vi "_allan_Variance_Ver6.vi"(6 "allan設定A":T1={"DMM設定A"={"間隔"=0.0001, "サンプルデータ数"=5000, "Voltage Range"=enum."1 V", "Factor"=1.0, "単位"=0, " 電源周波数(Hz)"=50.0}, "ファイルパス名"=path "c:/Data", "保存ファイル名"="", "DMM"=0, "DSA_mes"={"GPIB_DSA"="11", "Startfrq(Hz)"=0.0, "Stopfrq(Hz)"=800.0, "Range(Vpk)"=1.0, "average"=4}, " 温度？"=TRUE, "時間間隔（S）"=10.0} {"DMM" items=["DMM34410A", "34401A", "3458", "DSA35670A"]; "DMM設定A"."単位" items=["Sec", "PLC"]; "DMM設定A"."サンプルデータ数" min=1 max=1000000 step=1}) -> ()   [LabVIEW 2017]
uses:
  <vilib>/gmath/NI_Gmath.lvlib
panel:
  out "経過時間":dbl
  out "XYグラフ 4":cluster{"データ配列":dbl[], "データ配列":dbl[]}[](graph)
  out "配列":dbl[][](array[numeric])
  in  "終了時に機器を\nLOCAL":bool=TRUE
  out "FFT":cluster{dbl[], dbl[]}(graph)
  in  "計算を行う":bool=TRUE
  out "元データ":cluster{"時間":dbl[], "電圧":dbl[]}(graph)
  out "アラン分散":cluster{dbl[], dbl[]}(graph)
  # "アラン分散測定ソフト　Ver4\n　　ALMA-BAND4\n　　ALMA-BAND10"
  # "DMM      　 GPIB     　単位　　　　Factor　　　　　データ点数\n34410A  　23　　　　　　Sec　　　　　　１　　　　　　　MAX　50000\n34401A  　22　　　　　　PLC　　　　下記表参考　　MAX　512 \n3458　　　　22　　　　　　PLC　　　　下記表参考　　MAX 10240"
  # "facｔor　3458\nPLC=1 =>1\nPLC=0.1 => 1.0135\nPLC=0.01 => 1.1321"
  # "factor　３４４１０A \nPLCは以下から選択\nPLC=100　  　未確認\nPLC=10　  =>　1\nPLC=1 　   =>  1.03\nPLC=0.2 　 =>  0.83 \nPLC=0.02　 =>  1.714"
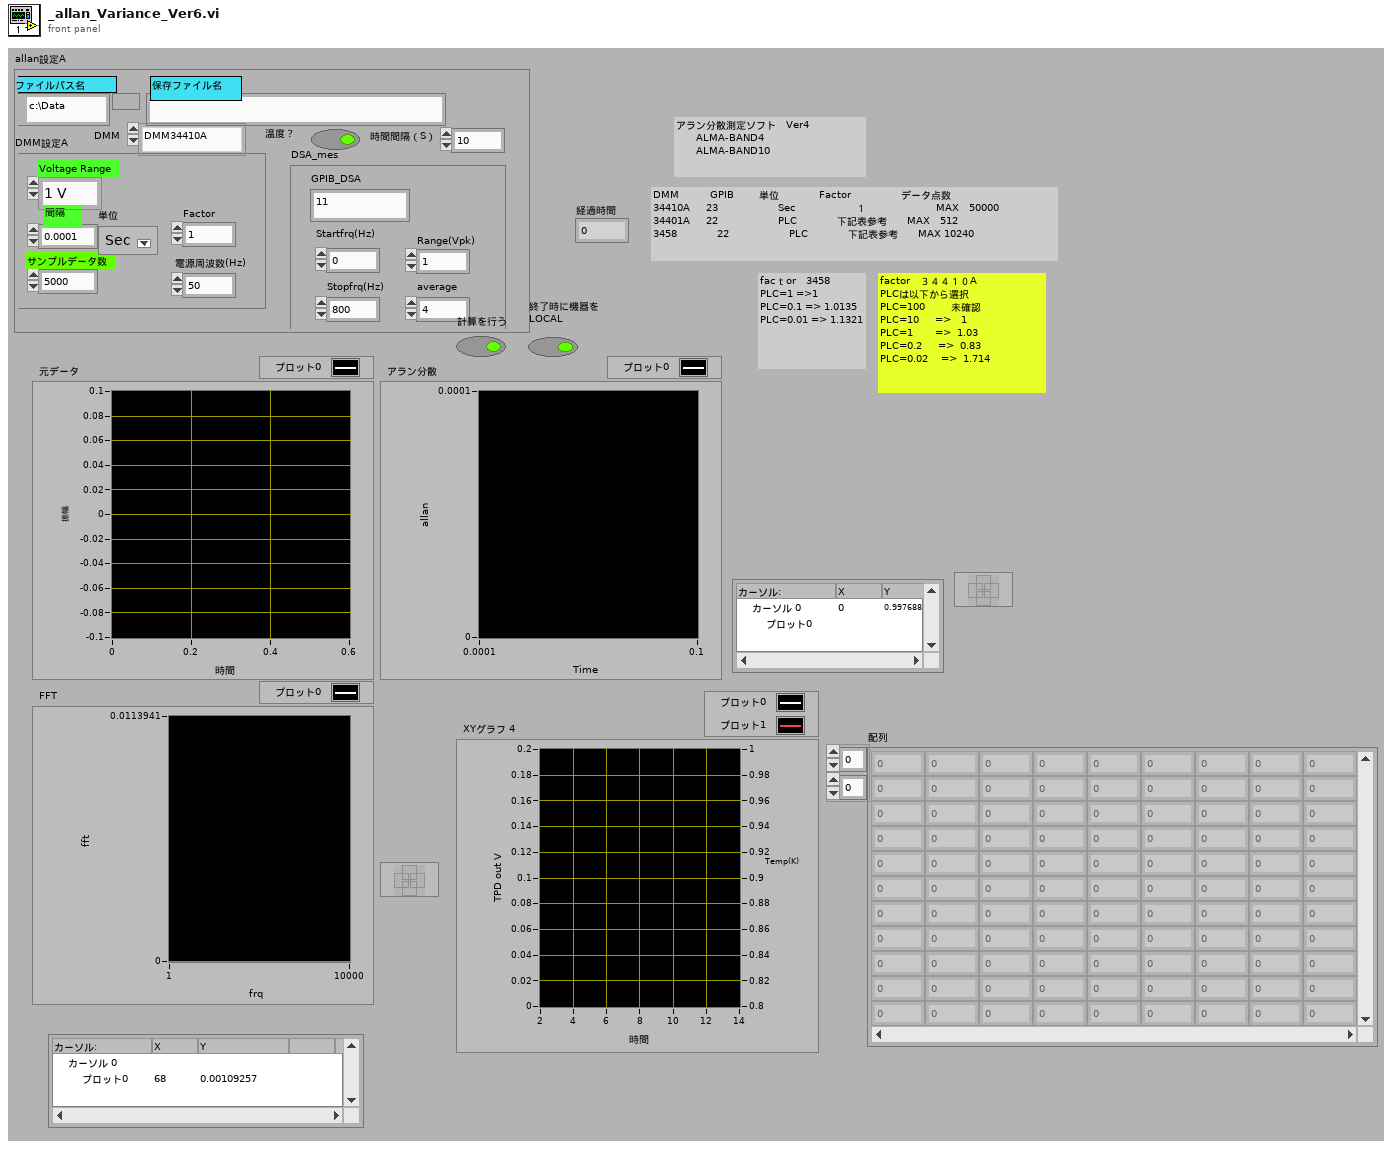
[diagram p1: front panel]
types:
  T1 = cluster{"DMM設定A":cluster{"間隔":dbl, "サンプルデータ数":i32, "Voltage Range":enum16{"100 mV", "1 V", "10 V", "100 V", "1000 V", "Auto", "Minimum", "Maximum"}, "Factor":dbl, "単位":u16, " 電源周波数(Hz)":dbl}, "ファイルパス名":path, "保存ファイル名":string, "DMM":u16, "DSA_mes":cluster{"GPIB_DSA":string, "Startfrq(Hz)":dbl, "Stopfrq(Hz)":dbl, "Range(Vpk)":dbl, "average":i16}, " 温度？":bool, "時間間隔（S）":dbl}
  T2 = cluster{"間隔":dbl, "サンプルデータ数":i32, "Voltage Range":enum16{"100 mV", "1 V", "10 V", "100 V", "1000 V", "Auto", "Minimum", "Maximum"}, "Factor":dbl, "単位":u16, " 電源周波数(Hz)":dbl}
  T3 = cluster{"GPIB_DSA":string, "Startfrq(Hz)":dbl, "Stopfrq(Hz)":dbl, "Range(Vpk)":dbl, "average":i16}
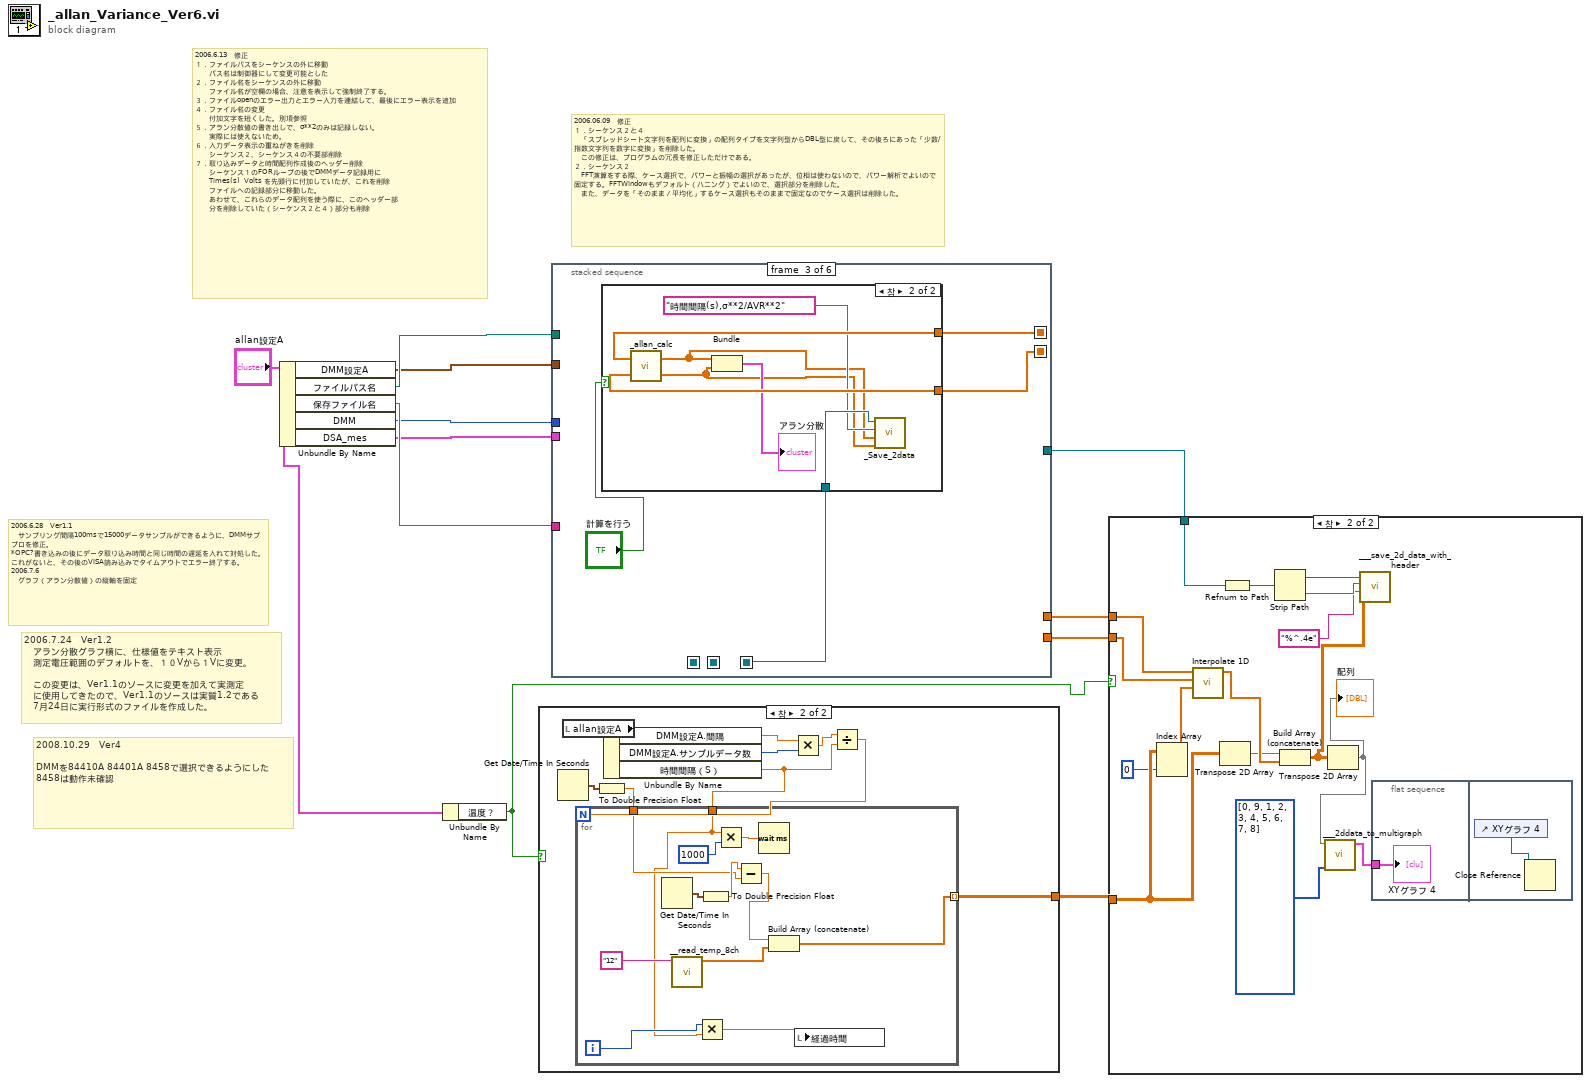
[diagram p0: block diagram]
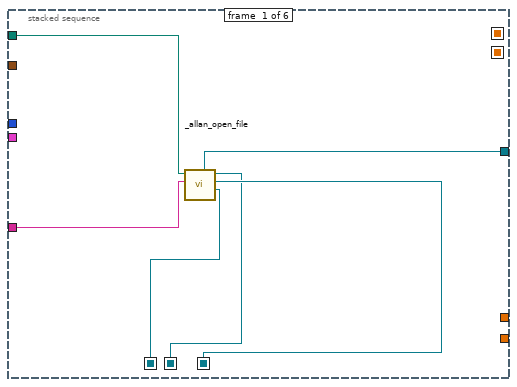
[diagram p4: hidden frame]
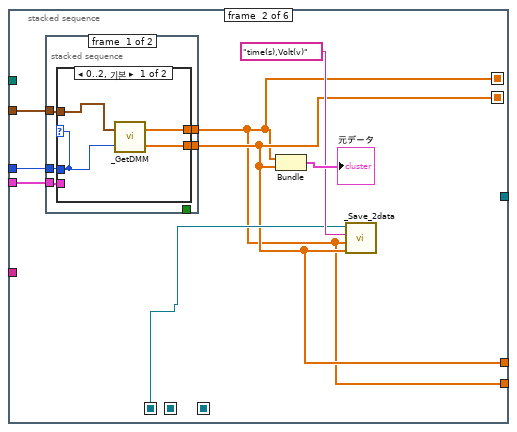
[diagram p5: hidden frame]
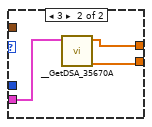
[diagram p6: hidden frame]
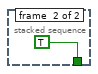
[diagram p7: hidden frame]
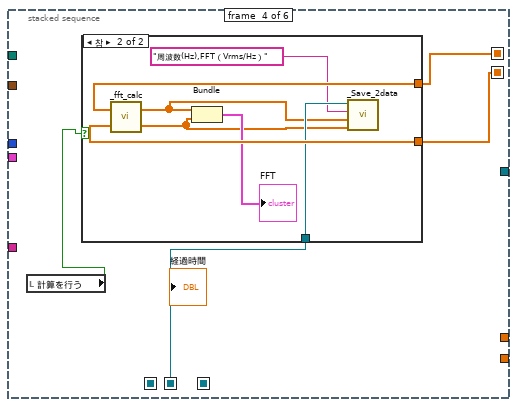
[diagram p9: hidden frame]
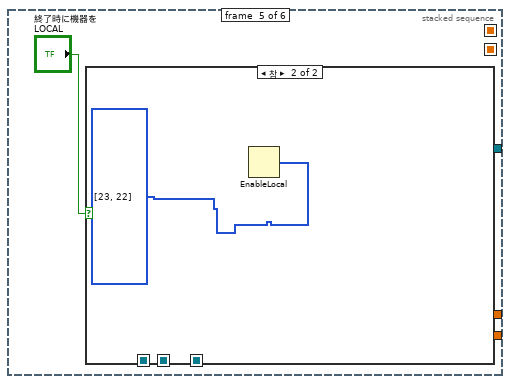
[diagram p11: hidden frame]
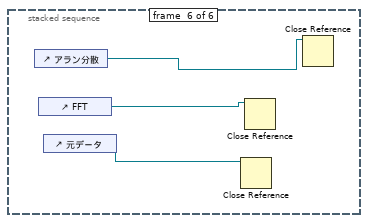
[diagram p13: hidden frame]
diagram:
  # "2008.10.29   Ver4 \n\nDMMを84410A 84401A 8458で選択できるようにした\n8458は動作未確認"
  # "2006.7.24   Ver1.2 \n　アラン分散グラフ横に、仕様値をテキスト表示\n　測定電圧範囲のデフォルトを、１０Vから１Vに変更。\n\n　この変更は、Ver1.1のソースに変更を加えて実測定\n　に使用してきたので、Ver1.1のソースは実質1.2である\n　7月24日に実行形式のファイルを作成した。"
  # "2006.6.28　Ver1.1\n　サンプリング間隔100msで15000データサンプルができるように、DMMサブプロを修正。\n*OPC?書き込みの後にデータ取り込み時間と同じ時間の遅延を入れて対処した。これがないと、その後のVISA読み込みでタイムアウトでエラー終了する。\n2006.7.6\n　グラフ（アラン分散値）の縦軸を固定"
  # "2006.6.13　修正\n１．ファイルパスをシーケンスの外に移動\n　　パス名は制御器にして変更可能とした\n２．ファイル名をシーケンスの外に移動\n　　ファイル名が空欄の場合、注意を表示して強制終了する。\n３．ファイルopenのエラー出力とエラー入力を連結して、最後にエラー表示を追加\n４．ファイル名の変更\n　　付加文字を短くした。別項参照\n５．アラン分散値の書き出しで、σ**2のみは記録しない。\n　　実際には使えないため。\n６．入力データ表示の重ねがきを削除\n　　シーケンス２、シーケンス４の不要部削除\n７．取り込みデータと時間配列作成後のヘッダー削除\n　　シーケンス１のFORループの後でDMMデータ記録用に\n　　Times(s)  Volts を先頭行に付加していたが、これを削除\n　　ファイルへの記録部分に移動した。\n　　あわせて、これらのデータ配列を使う際に、このヘッダー部\n　　分を削除していた（シーケンス２と４）部分も削除"
  # "2006.06.09　修正\n１．シーケンス２と４\n　「スプレッドシート文字列を配列に変換」の配列タイプを文字列型からDBL型に戻して、その後ろにあった「少数/指数文字列を数字に変換」を削除した。\n　この修正は、プログラムの冗長を修正しただけである。\n２．シーケンス２\n　FFT演算をする際、ケース選択で、パワーと振幅の選択があったが、位相は使わないので、パワー解析でよいので固定する。FFTWindowもデフォルト（ハニング）でよいので、選択部分を削除した。\n　また、データを「そのまま／平均化」するケース選択もそのままで固定なのでケース選択は削除した。"
  n1 = Unbundle By Name("allan設定A") -> ("DMM設定A"=w9:T2, "ファイルパス名"=w11:path, "保存ファイル名"=w10:string, "DMM"=w8:u16, "DSA_mes"=w7:T3)
  n2 = Unbundle By Name("allan設定A") -> ("温度？"=w5:bool)
  n3 = case shown="참" w5 {
    tunnel: [_ w12] -> w2
    frame False {
    }
    frame True {
      n4 = Get Date/Time In Seconds() -> (seconds since 1Jan1904=w14:timestamp)
      n5 = local read "allan設定A"() -> (w20:T1)
      n6 = To Double Precision Float(number=w14) -> (double precision float=w13:dbl)
      n7 = Unbundle By Name(w20) -> ("DMM設定A.間隔"=w19:dbl, "DMM設定A.サンプルデータ数"=w18:i32, "時間間隔（S）"=w15:dbl)
      n8 = Multiply(x=w19, y=w18) -> (x*y=w17:dbl)
      n9 = Divide(x=w17, y=w15) -> (x/y=w16:dbl)
      n10 = for {
        N: w16 -> [_]
        tunnel: [w31] -> w12 mode=indexing
        tunnel: w15 -> [w22]
        tunnel: w13 -> [w27]
        i -> [w23]
        n11 = Get Date/Time In Seconds() -> (seconds since 1Jan1904=w32:timestamp)
        n12 = call "__read_temp_8ch.vi"("GIPB番号"="12") -> ("配列"=w25:dbl[])  [unwired: 10 in]
        n13 = Multiply(x=w23, y=w22) -> (x*y=w21:dbl)
        n14 = To Double Precision Float(number=w32) -> (double precision float=w28:dbl)
        n15 = Multiply(x=w22, y=1000) -> (x*y=w29:dbl)
        n16 = Subtract(x=w28, y=w27) -> (x-y=w26:dbl)
        n17 = Wait (ms)(milliseconds to wait=w29) -> ()  [unwired: 1 out]
        n18 = Build Array (concatenate)(w26, w25) -> (w31:dbl[])
        n19 = local write "経過時間"(w21) -> ()
      }
    }
  }
  n20 = stacked-sequence {
    seq-local: [w38 _ _ _ _ _] -> [_ w41 _ _ _ _]
    seq-local: [_ w39 _ _ _ _] -> [_ _ w63 w74 _ _]
    seq-local: [w37 _ _ _ _ _] -> [_ _ w61 _ _ _]
    seq-local: [w36 _ _ _ _ _] -> [_ _ _ w72 _ _]
    seq-local: [_ w40 _ _ _ _] -> [_ _ w62 w73 _ _]
    tunnel: w11 -> [w34 _ _ _ _ _]
    tunnel: w10 -> [w35 _ _ _ _ _]
    tunnel: w9 -> [_ w45 _ _ _ _]
    tunnel: w8 -> [_ w43 _ _ _ _]
    tunnel: w7 -> [_ w42 _ _ _ _]
    tunnel: [_ w40 _ _ _ _] -> w4
    tunnel: [_ w39 _ _ _ _] -> w3
    tunnel: [w33 _ _ _ _ _] -> w1
    frame #0 {
      n21 = call "_allan_open_file.vi"("保存ファイル名"=w35, "ファイルパス名"=w34) -> ("refnum data"=w38:refnum<file>, "refnum allan"=w37:refnum<file>, "refnum_fft"=w36:refnum<file>, "refnum temp"=w33:refnum<file>)  [unwired: 3 in, 1 out]
    }
    frame #1 {
      n22 = stacked-sequence {
        tunnel: w45 -> [w51 _]
        tunnel: [w50 _] -> w39
        tunnel: [w49 _] -> w40
        tunnel: w43 -> [w48 _]
        tunnel: w42 -> [w47 _]
        tunnel: [_ TRUE] -> _
        frame #0 {
          n23 = case shown="0..2, 기본" w48 {
            tunnel: w51 -> [w55 _]
            tunnel: w48 -> [w54 _]
            tunnel: [w53 w57] -> w50
            tunnel: [w52 w56] -> w49
            tunnel: w47 -> [_ w58]
            frame 0..2, Default {
              n24 = call "_GetDMM.vi"("DMM"=w54, "DMM設定A"=w55) -> ("電圧"=w52:dbl[], "時間"=w53:dbl[])
            }
            frame 3 {
              n25 = call "__GetDSA_35670A.vi"("DSA_mes"=w58) -> ("電圧"=w56:dbl[], "時間"=w57:dbl[])  [unwired: 9 in]
            }
          }
        }
        frame #1 {
        }
      }
      n26 = Bundle("時間"=w39, "電圧"=w40) -> (→"元データ":cluster{"時間":dbl[], "電圧":dbl[]})  [unwired: 1 in]
      n27 = call "_Save_2data.vi"("データ2"=w40, "データ1"=w39, "項目名称"="time(s),Volt(v)", "refnum"=w41) -> ()  [unwired: 4 in]
    }
    frame #2 {
      n28 = case shown="참" "計算を行う" {
        tunnel: w63 -> [_ w70]
        tunnel: w62 -> [_ w69]
        tunnel: w61 -> [_ w67]
        frame False {
        }
        frame True {
          n29 = call "_allan_calc.vi"("電圧"=w69, "時間"=w70) -> ("アラン分散"=w64:dbl[], "アラン時間"=w65:dbl[])
          n30 = Bundle("アラン時間"=w65, "アラン分散"=w64) -> (→"アラン分散":cluster{"アラン時間":dbl[], "アラン分散":dbl[]})  [unwired: 1 in]
          n31 = call "_Save_2data.vi"("データ2"=w64, "データ1"=w65, "項目名称"="時間間隔(s),σ**2/AVR**2", "refnum"=w67) -> ()  [unwired: 4 in]
        }
      }
    }
    frame #3 {
      n32 = local read "計算を行う"() -> (w71:bool)
      n33 = case shown="참" w71 {
        tunnel: w74 -> [_ w81]
        tunnel: w73 -> [_ w80]
        tunnel: w72 -> [_ w78]
        frame False {
        }
        frame True {
          n34 = call "_fft_calc.vi"("電圧"=w80, "時間"=w81) -> ("FFTパワー"=w76:dbl[], "FFT周波数"=w77:dbl[])
          n35 = Bundle("FFT周波数"=w77, "FFTパワー"=w76) -> (→"FFT":cluster{"FFT周波数":dbl[], "FFTパワー":dbl[]})  [unwired: 1 in]
          n36 = call "_Save_2data.vi"("データ2"=w76, "データ1"=w77, "項目名称"="周波数(Hz),FFT（Vrms/Hz）", "refnum"=w78) -> ()  [unwired: 4 in]
        }
      }
    }
    frame #4 {
      n37 = case shown="참" "終了時に機器を\nLOCAL" {
        frame False {
        }
        frame True {
          n38 = EnableLocal(3:i32[] [23, 22]) -> ()  [unwired: 2 in, 2 out]
        }
      }
    }
    frame #5 {
      n39 = control-ref of="アラン分散"() -> (w86:refnum<vi>)
      n40 = control-ref of="FFT"() -> (w85:refnum<vi>)
      n41 = control-ref of="元データ"() -> (w84:refnum<vi>)
      n42 = Close Reference(reference=w84) -> ()  [unwired: 1 in, 1 out]
      n43 = Close Reference(reference=w85) -> ()  [unwired: 1 in, 1 out]
      n44 = Close Reference(reference=w86) -> ()  [unwired: 1 in, 1 out]
    }
  }
  n45 = case shown="참" w5 {
    tunnel: w4 -> [_ w102]
    tunnel: w3 -> [_ w101]
    tunnel: w2 -> [_ w99]
    tunnel: w1 -> [_ w93]
    frame False {
    }
    frame True {
      n46 = Index Array(array=w99, index (col)=0) -> (element=w100:dbl[])  [unwired: 1 in]
      n47 = call <vilib>:"Interpolate 1D.vi"("xi"=w100, "X"=w101, "Y"=w102) -> ("yi"=w98:dbl[])  [unwired: 6 in, 2 out]
      n48 = Transpose 2D Array(2D array=w99) -> (transposed array=w96:dbl[][])
      n49 = Refnum to Path(1:w93) -> (0:w92:path)
      n50 = Strip Path(path=w92) -> (stripped path=w91:path, name=w90:string)
      n51 = Build Array (concatenate)(w96, w98) -> (w87:dbl[][])
      n52 = Transpose 2D Array(2D array=w87) -> (transposed array=w89:dbl[][])
      "配列" <- w89
      n53 = call "___2ddata_to_multigraph.vi"("列"=i32[] [0, 9, 1, 2, 3, 4, 5, 6, 7, 8], "データ配列"=w89) -> ("XYグラフ"=w94:cluster{"データ配列":dbl[], "データ配列":dbl[]}[])  [unwired: 5 in]
      n54 = call "___save_2d_data_with_header.vi"("配列"=w87, "形式"="%^.4e", "file_name"=w90, "パス"=w91) -> ()  [unwired: 7 in, 1 out]
      n55 = flat-sequence {
        tunnel: w94 -> [w103]
        frame #0 {
          "XYグラフ 4" <- w103
        }
        frame #1 {
          n56 = control-ref of="XYグラフ 4"() -> (w104:refnum<vi>)
          n57 = Close Reference(reference=w104) -> ()  [unwired: 1 in, 1 out]
        }
      }
    }
  }
